vi "Load INI Config_EStop.vi"(8 "error in":errorcluster, 11 "configuration file path":path) -> (0 "error out":errorcluster)   [LabVIEW 2021]
uses:
  DAQ_Data.ctl
  Measure Type.ctl
  MUX_Data.ctl
  DMM_Data.ctl
  <vilib>/Utility/config.llb/Read Key (String).vi
  <vilib>/Utility/config.llb/NI_LVConfig.lvlib
panel:
  out "data":T1[](array[typedef])
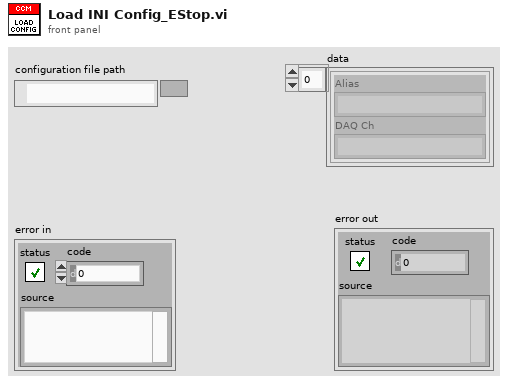
[diagram p1: front panel]
types:
  T1 = typedef "DAQ_Data.ctl" = cluster{"Alias":string, "DAQ Ch":string}
  T2 = typedef "NI_LVConfig.lvlib/Config Data RefNum.ctl" = refnum<k1>
  T3 = typedef "MUX_Data.ctl" = cluster{"Channel":string, "Topology":string}
  T4 = typedef "DMM_Data.ctl" = cluster{"Channel":string, "MUX":string, "Route":string}
  T5 = typedef "Measure Type.ctl" = enum16{"Analog In", "Analog Out", "Digital In", "Digital Out", "Switch", "NI DMM"}
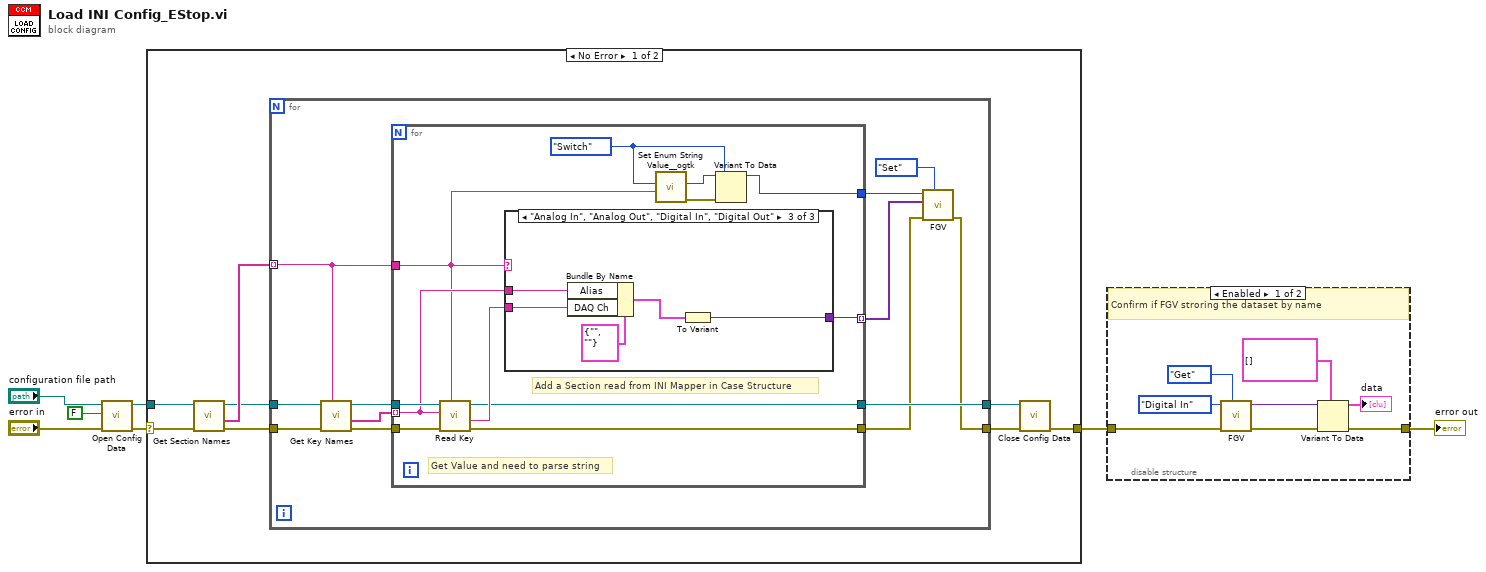
[diagram p0: block diagram]
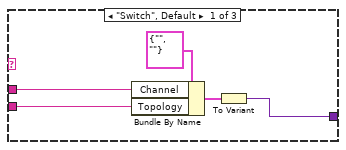
[diagram p2: hidden frame]
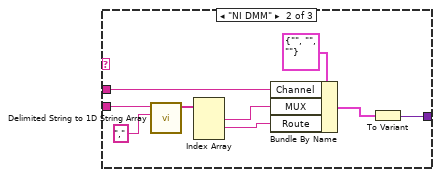
[diagram p3: hidden frame]
diagram:
  n1 = call <vilib>:"Open Config Data.vi"("error in (no error)"="error in", "create file if necessary (T)"=FALSE, "configuration file path"="configuration file path") -> ("error out"=w5:errorcluster, "refnum"=w6:T2)  [unwired: 6 in, 1 out]
  n2 = case shown="No Error" w5 {
    selector: w5 -> [w15 w59]
    tunnel: [w8 w59] -> w3
    tunnel: w6 -> [w14 _]
    frame No Error {
      n3 = call <vilib>:"Get Section Names.vi"("error in (no error)"=w15, "refnum"=w14) -> ("error out"=w12:errorcluster, "section names"=w13:string[], "refnum out"=w11:T2)  [unwired: 7 in]
      n4 = for {
        tunnel: w13 -> [w24] mode=indexing
        tunnel: w12 -> [w27]
        tunnel: w11 -> [w26]
        tunnel: [w25] -> w10
        tunnel: [w17] -> w9
        n5 = call <vilib>:"Get Key Names.vi"("section"=w24, "error in (no error)"=w27, "refnum"=w26) -> ("error out"=w23:errorcluster, "key names"=w22:string[], "refnum out"=w21:T2)  [unwired: 5 in, 1 out]
        n6 = for {
          tunnel: w23 -> [w39]
          tunnel: w22 -> [w36] mode=indexing
          tunnel: w24 -> [w30]
          tunnel: w21 -> [w38]
          tunnel: [w34] -> w25
          tunnel: [w37] -> w18
          tunnel: [w33] -> w19 mode=indexing
          tunnel: [w29] -> w16
          w28 = Measure_Type."Switch" ("Name")
          # "Add a Section read from INI Mapper in Case Structure"
          # "Get Value and need to parse string"
          n7 = call-poly <vilib>:"Read Key.vi"("section"=w30, "error in (no error)"=w39, "key"=w36, "refnum"=w38) -> ("error out"=w37:errorcluster, "value"=w35:string, "refnum out"=w34:T2)  [unwired: 4 in, 1 out]
          n8 = case shown="\"Analog In\", \"Analog Out\", \"Digital In\", \"Digital Out\"" w30 {
            tunnel: w36 -> [w43 w47 w56]
            tunnel: w35 -> [w42 w50 w55]
            tunnel: [w41 w48 w58] -> w33
            frame "Switch", Default {
              n9 = Bundle By Name(cluster=T3 {"Channel"="", "Topology"=""}, "Channel"=w43, "Topology"=w42) -> (w40:T3)
              n10 = To Variant(anything=w40) -> (Variant=w41:variant)
            }
            frame "NI DMM" {
              n11 = call <vilib>:"Delimited String to 1D String Array.vi"("delimiter"=",", "delimited string"=w50) -> ("string array"=w52:string[])  [unwired: 9 in]
              n12 = Index Array(array=w52) -> (element #1=w46:string, element #2=w45:string)  [unwired: 3 in, 1 out]
              n13 = Bundle By Name(cluster=T4 {"Channel"="", "MUX"="", "Route"=""} ("DAQ Data"), "Channel"=w47, "MUX"=w46, "Route"=w45) -> (w49:T4)
              n14 = To Variant(anything=w49) -> (Variant=w48:variant)
            }
            frame "Analog In", "Analog Out", "Digital In", "Digital Out" {
              n15 = Bundle By Name(cluster=T1 {"Alias"="", "DAQ Ch"=""} ("DAQ Data"), "Alias"=w56, "DAQ Ch"=w55) -> (w54:T1)
              n16 = To Variant(anything=w54) -> (Variant=w58:variant)
            }
          }
          n17 = call <userlib>:"Set Enum String Value__ogtk.vi"("String Value"=w30, "Default Enum Value"=w28) -> ("error out"=w32:errorcluster, "Enum"=w31:variant)  [unwired: 8 in]
          n18 = Variant To Data(error in=w32, type=w28, Variant=w31) -> (data=w29:T5)  [unwired: 1 out]
        }
        n19 = call "FGV.vi"("Method (Get)"=enum16{"Get", "Set"}."Set", "error in"=w18, "Data In"=w19, "Name"=w16) -> ("error out"=w17:errorcluster)  [unwired: 6 in, 1 out]
      }
      n20 = call <vilib>:"Close Config Data.vi"("error in (no error)"=w9, "refnum"=w10) -> ("error out"=w8:errorcluster)  [unwired: 8 in, 1 out]
    }
    frame Error {
    }
  }
  n21 = disable-structure shown="Enabled" {
    disable-tunnel: w3 -> [w67 w68]
    disable-tunnel: [w63 w68] -> w2
    frame Enabled {
      # "Confirm if FGV stroring the dataset by name"
      n22 = call "FGV.vi"("Method (Get)"=enum16{"Get", "Set"}."Get", "error in"=w67, "Name"=Measure_Type."Digital In") -> ("error out"=w65:errorcluster, "Data out"=w64:variant)  [unwired: 7 in]
      n23 = Variant To Data(error in=w65, type=T1[] [], Variant=w64) -> (data=→"data":T1[], error out=w63:errorcluster)
    }
    frame Disabled {
    }
  }
  "error out" <- w2
